vi "test Queue ACL.vi"(8 "error in (no error)":errorcluster, 11 "TestCase in":refnum<class "Test_Queue.lvclass">) -> (0 "error out":errorcluster, 3 "TestCase out":refnum<class "Test_Queue.lvclass">)   [LabVIEW 2015, in "Test_Queue.lvclass"]
uses:
  Test_Queue.lvclass
  Queue/Signed Identifier.ctl
  Queue/Access Policy.ctl
  Global Parameters.vi
  Core/Session/Session.lvclass
  Queue/NI_Azure_Queue.lvlib
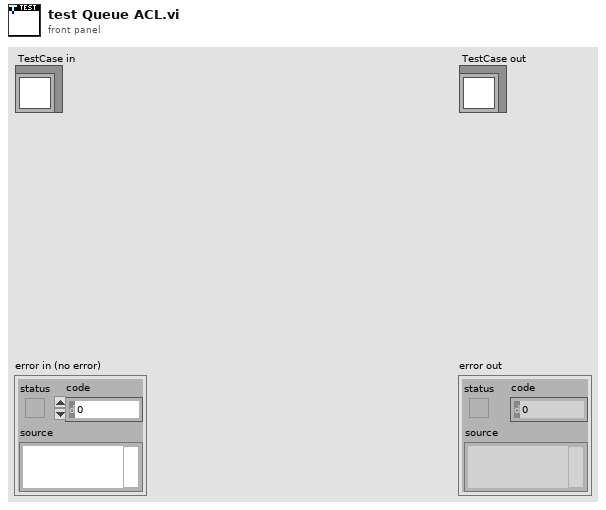
[diagram p1: front panel]
types:
  T1 = typedef "NI_Azure_Queue.lvlib/Signed Identifier.ctl" = cluster{"ID":string, "Access policy":T2}
  T2 = typedef "NI_Azure_Queue.lvlib/Access Policy.ctl" = cluster{"Start":string, "Expiry":string, "Permission":string}
  T3 = typedef "NI_Azure_Core.lvlib/Azure Credentials.ctl" = cluster{"Storage Account Name":string, "Access Key":string}
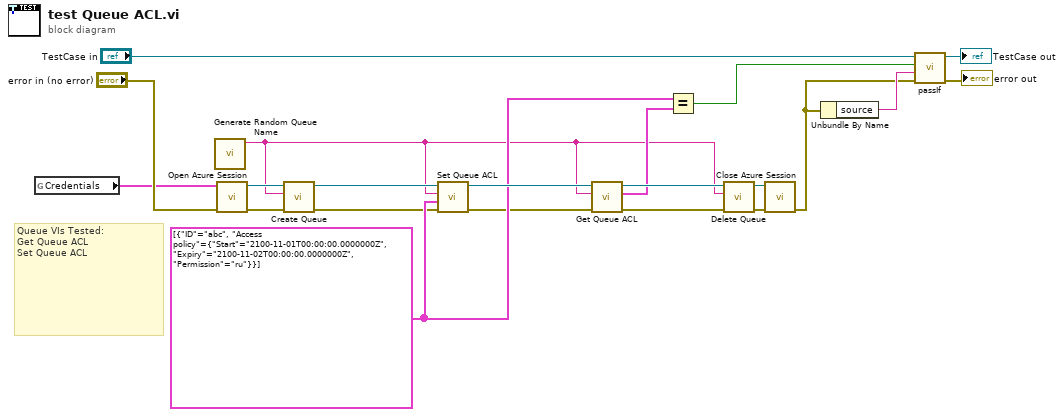
[diagram p0: block diagram]
diagram:
  w4 = T1[] [{"ID"="abc", "Access policy"={"Start"="2100-11-01T00:00:00.0000000Z", "Expiry"="2100-11-02T00:00:00.0000000Z", "Permission"="ru"}}] ("ACL")
  # "Queue VIs Tested:\nGet Queue ACL\nSet Queue ACL"
  n1 = global read "Global Parameters.vi" "Credentials"() -> (w15:T3)
  n2 = call "Generate Random Queue Name.vi"() -> ("Random Queue Name"=w1:string)  [unwired: 11 in]
  n3 = call "Open Azure Session.vi"("error in (no error)"="error in (no error)", "Credentials"=w15) -> ("error out"=w16:errorcluster, "Azure Session"=w13:refnum<class "Session.lvclass">)  [unwired: 8 in]
  n4 = call "Create Queue.vi"("error in (no error)"=w16, "Queue"=w1, "Azure Session in"=w13) -> ("error out"=w3:errorcluster, "Azure Session out"=w8:refnum<class "Session.lvclass">)  [unwired: 7 in]
  n5 = call "Set Queue ACL.vi"("error in (no error)"=w3, "ACL"=w4, "Queue"=w1, "Azure Session in"=w8) -> ("error out"=w2:errorcluster, "Azure Session out"=w7:refnum<class "Session.lvclass">)  [unwired: 6 in]
  n6 = call "Get Queue ACL.vi"("error in (no error)"=w2, "Queue"=w1, "Azure Session in"=w7) -> ("error out"=w10:errorcluster, "ACL"=w5:T1[], "Azure Session out"=w9:refnum<class "Session.lvclass">)  [unwired: 6 in]
  n7 = Equal?(x=w4, y=w5) -> (x = y?=w6:bool)
  n8 = call "Delete Queue.vi"("error in (no error)"=w10, "Queue"=w1, "Azure Session in"=w9) -> ("error out"=w14:errorcluster, "Azure Session out"=w12:refnum<class "Session.lvclass">)  [unwired: 7 in]
  n9 = call "Close Azure Session.vi"("error in (no error)"=w14, "Azure Session"=w12) -> ("error out"=w11:errorcluster)  [unwired: 9 in]
  n10 = Unbundle By Name(w11) -> ("source"=w18:string)
  n11 = call-dynamic "passIf.vi"("error in (no error)"=w11, "message (\"\")"=w18, "pass"=w6, "TestCase in"="TestCase in") -> ("error out"=→"error out":errorcluster, "TestCase out"=→"TestCase out":refnum<class "Test_Queue.lvclass">)  [unwired: 6 in]
